vi "CHANNEL_CFG.vi"(1 "error in (no error)":errorcluster, 2 "VISA resource name":refnum<visa-resource-name>, 4 "Channel":dbl=2.0, 5 "Mode":dbl, 6 "Gain":dbl=3.0, 7 "Nchan":dbl=1.0, 8 "Pchan":dbl=1.0) -> (0 "error out":errorcluster, 3 "VISA resource name out":refnum<visa-resource-name>)   [LabVIEW 2011]
panel:
  out "unsigned byte array":u8[](array[numeric])
  out "return count":u32
  out "Read Channel_CFG":u8[](array[numeric])
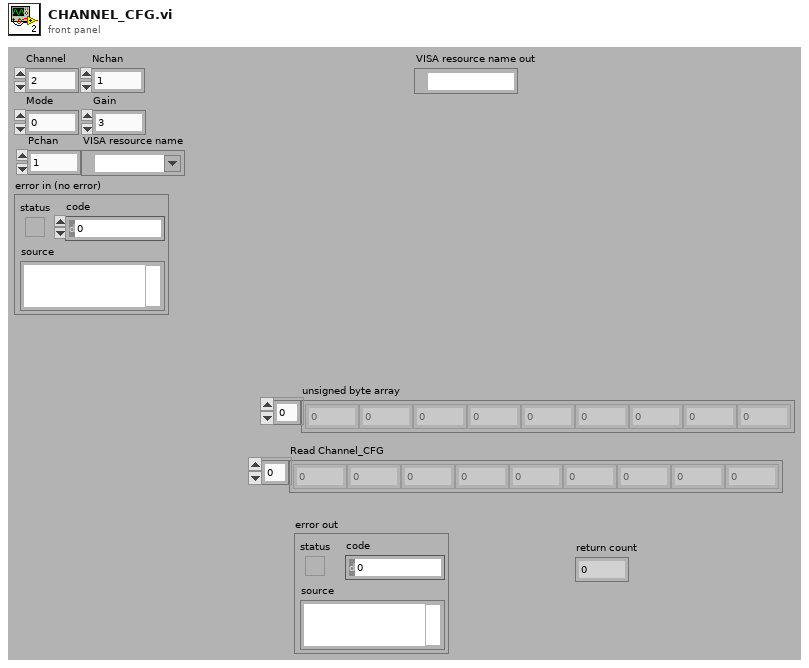
[diagram p1: front panel]
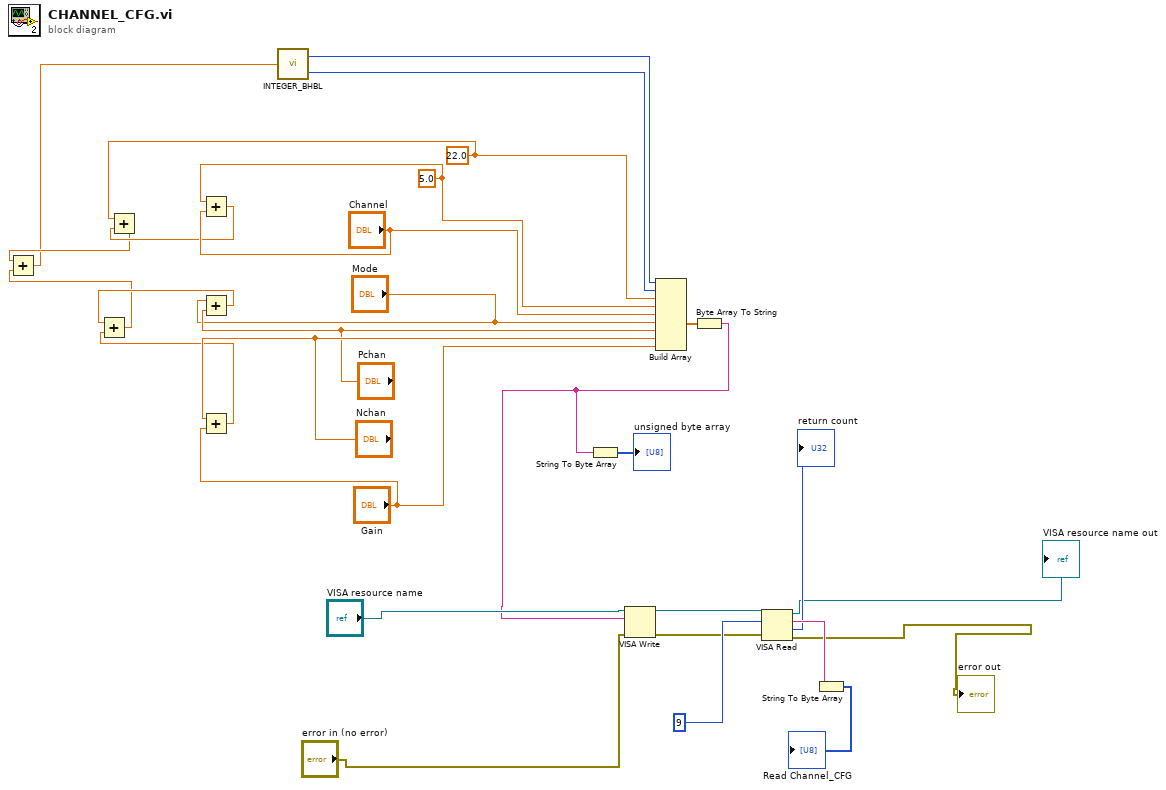
[diagram p0: block diagram]
diagram:
  w10 = 5.0 ("element")
  w8 = 22.0 ("element")
  n1 = Add(x=w10, y="Channel") -> (x+y=w9:dbl)
  n2 = Add(x=w8, y=w9) -> (x+y=w7:dbl)
  n3 = Add(x="Mode", y="Pchan") -> (x+y=w12:dbl)
  n4 = Add(x="Nchan", y="Gain") -> (x+y=w15:dbl)
  n5 = Add(x=w12, y=w15) -> (x+y=w6:dbl)
  n6 = Add(x=w7, y=w6) -> (x+y=w5:dbl)
  n7 = call "INTEGER_BHBL.vi"("int16"=w5) -> ("Lvalue"=w3:u8, "HValue"=w4:u8)
  n8 = Build Array(w4, w3, w8, w10, "Channel", "Mode", "Pchan", "Nchan", "Gain") -> (w23:dbl[])
  n9 = Byte Array To String(unsigned byte array=w23) -> (string=w2:string)
  n10 = String To Byte Array(string=w2) -> (unsigned byte array=→"unsigned byte array":u8[])
  n11 = VISA Write(VISA resource name="VISA resource name", write buffer=w2, error in (no error)="error in (no error)") -> (VISA resource name out=w24:refnum<visa-resource-name>, error out=w25:errorcluster)  [unwired: 1 out]
  n12 = VISA Read(VISA resource name=w24, byte count=u32 9, error in (no error)=w25) -> (VISA resource name out=→"VISA resource name out":refnum<visa-resource-name>, read buffer=w27:string, return count=→"return count":u32, error out=→"error out":errorcluster)
  n13 = String To Byte Array(string=w27) -> (unsigned byte array=→"Read Channel_CFG":u8[])
